vi "TestLauncher.vi"() -> ()   [LabVIEW 2020, in "ECU_Diagnose.lvlib"]
uses:
  ECU_Diagnose.lvlib
  SignalSenderLoop/SignalSenderLoop.lvclass
  C:/Program Files (x86)/National Instruments/LabVIEW 2020/vi.lib/JKI/JKI SMO/SMO/SMO.lvclass
  SignalReceiver/Typedefs/SignalArrySelecte.ctl
  SignalSenderLoop/subvi/SignalFrameSet.ctl
  SignalReceiver/GlobalData_operation.ctl
  SignalReceiver/SignalReceiver.lvclass
  <vilib>/JKI/JKI SMO/SMO/SMO.lvclass
  UDS_class/UDS.lvclass
  <vilib>/addons/_AddQ/G#Object/G#Object.lvclass
  <vilib>/Automotive Diagnostic Command Set/Diagnostic Transport.llb/Property ID.ctl
  <vilib>/addons/Automotive Diagnostic Command Set/NI_Automotive Diagnostic Command Set.lvlib
  <vilib>/Utility/config.llb/NI_LVConfig.lvlib
panel:
  in  "ClaerData":bool
  in  "Close":bool
  in  "总关闭":bool
  in  "信号收发参数":T3={"信号接收参数"={"Port_No."="CAN1", "XNET Signal"=[]}, "信号轮询发送参数"={"XNET SignalFrameArry"=[{"Port_No."="CAN1", "计数Count"=TRUE, "校验CheckSum"=TRUE, "MessageFrame"="ESP_1\nLR110", "校验算法名称"="Anti_Add"}, {"Port_No."="CAN1", "计数Count"=FALSE, "校验CheckSum"=FALSE, "MessageFrame"="VTOG_1\nLR110", "校验算法名称"=""}]}}
  in  "Save":bool
  in  "Read":bool
  out "DataIdentify":string
  out "Clear DTC":bool
  out "DID":u8[](array[numeric]) format="%.0x"
  out "OK":bool
  out "# of objects killed":i32
  out "Waveform Graph":dbl[][](graph)
  in  "StartStop":bool
  in  "Stop 2":bool
  out "error out":errorcluster
  out "数组":errorcluster[](array[cluster])
  in  "SignalsSet":dbl[](array[numeric])=[-32.0, 0.0, 1.0, 0.0, 1.0, 0.0, 1.0, 0.0, 1.0, 0.0, 1.0, 0.0, 1.0]
  in  "Stop":bool
  in  "SignalsSet 2":dbl[](array[numeric])=[0.0]
  out "元素":refnum<class "SignalSenderLoop.lvclass">
  out "SMOArry":refnum<class "SignalSenderLoop.lvclass">[](array[class])
  # "Signals Sender"
  # "数组为空，不发送任何帧，即停止发送\n首次运行时需要值改变触发一下"
  # "Signals Receiver"
  # "UDS Dignose Sender"
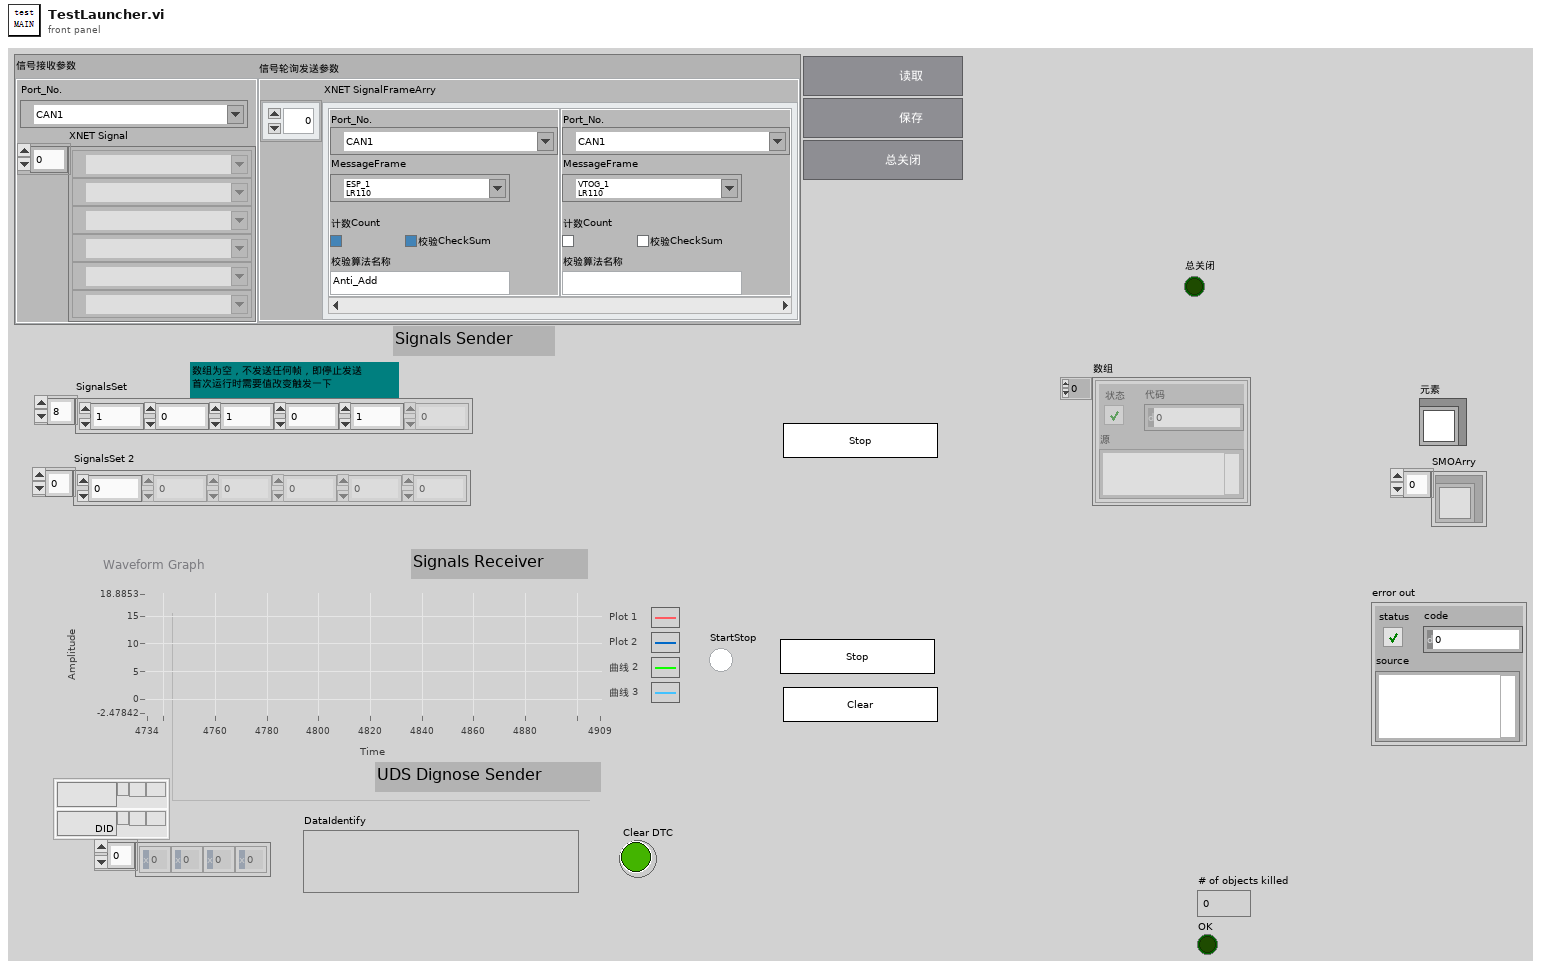
[diagram p1: front panel]
types:
  T1 = typedef "ECU_Diagnose.lvlib/SignalReceiver.lvclass/SignalArrySelecte.ctl" = cluster{"Port_No.":refnum<k21>, "XNET Signal":refnum<k21>[]}
  T2 = typedef "ECU_Diagnose.lvlib/SignalSenderLoop.lvclass/SignalFrameSet.ctl" = cluster{"Port_No.":refnum<k21>, "计数Count":bool, "校验CheckSum":bool, "MessageFrame":refnum<k21>, "校验算法名称":string}
  T3 = cluster{"信号接收参数":T1, "信号轮询发送参数":cluster{"XNET SignalFrameArry":T2[]}}
  T4 = typedef "GlobalData_operation.ctl" = enum16{"idle", "read", "write", "clear", "init", "destroy"}
  T5 = typedef "NI_Automotive Diagnostic Command Set.lvlib/Property ID.ctl" = enum16{"Timeout Diag Command", "Timeout FC (Bs)", "Timeout CF (Cr)", "Receive Block Size (BS)", "Wait Time CF (STmin)", "Max Wait Frames (N_WFTmax)", "Wait Frames to Send (N_WAIT)", "Time between Waits (T_W)", "Fill CAN Frames", "Fill Byte", "Invalid Response as Error", "Max RspPending Count", "VWTP Command Timeout", "STmin", "P2min", "Termination", "Timeout RspPending", "LIN Sleep", "Actual CAN IO Mode", "Response Plausibility Check", "Session-based Properties"}
  T6 = typedef "NI_LVConfig.lvlib/Config Data RefNum.ctl" = refnum<k1>
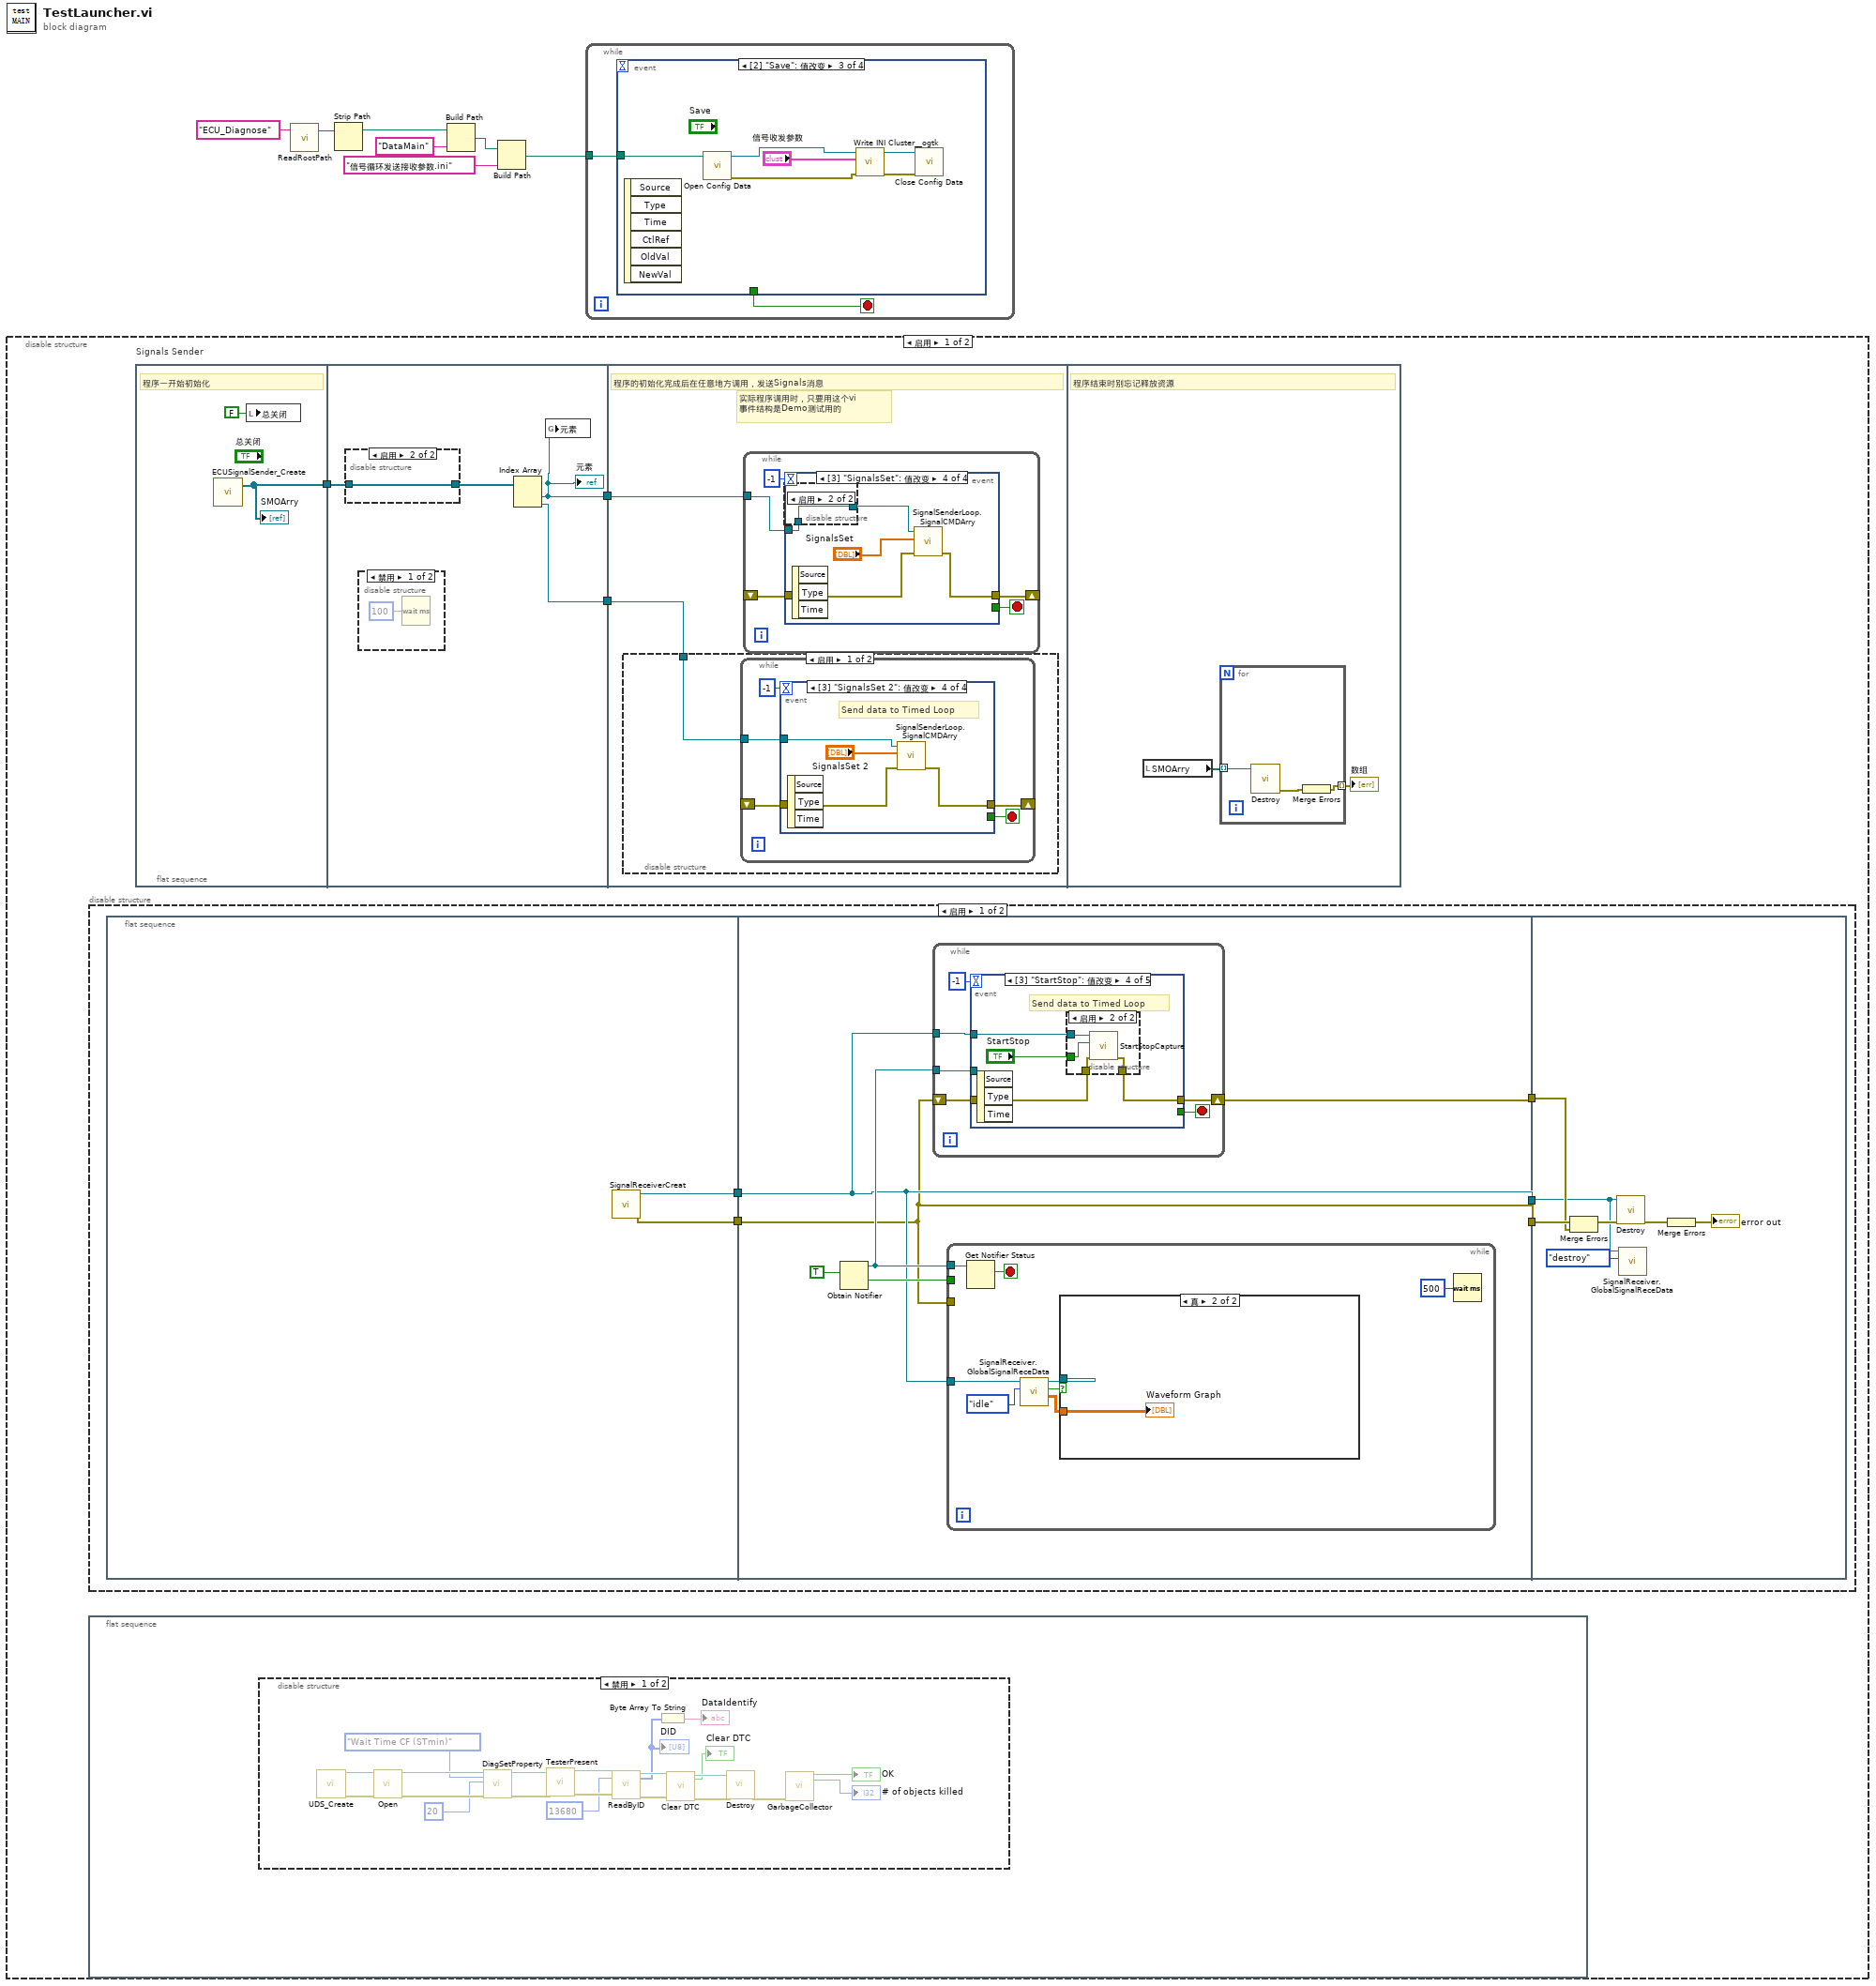
[diagram p0: block diagram]
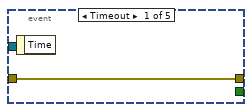
[diagram p3: hidden frame]
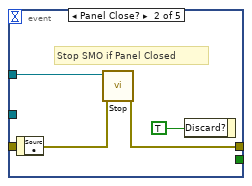
[diagram p4: hidden frame]
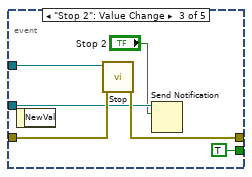
[diagram p5: hidden frame]
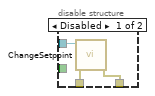
[diagram p6: hidden frame]
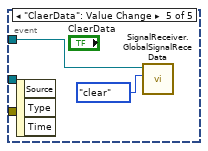
[diagram p7: hidden frame]
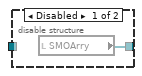
[diagram p10: hidden frame]
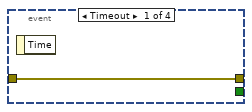
[diagram p12: hidden frame]
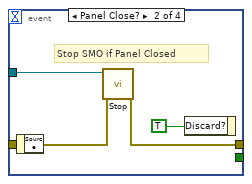
[diagram p13: hidden frame]
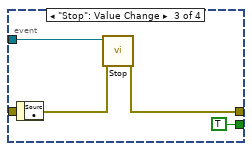
[diagram p14: hidden frame]
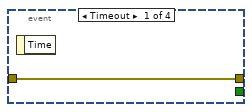
[diagram p16: hidden frame]
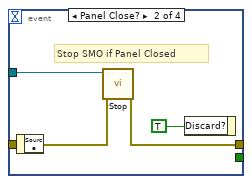
[diagram p17: hidden frame]
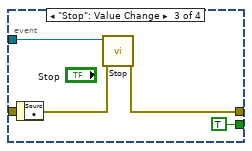
[diagram p18: hidden frame]
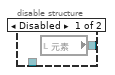
[diagram p19: hidden frame]
diagram:
  n1 = disable-structure shown="启用" {
    frame Enabled {
      n2 = flat-sequence {
        frame #0 {
          n3 = disable-structure shown="禁用" {
            frame Disabled {
              n4 = call "UDS_Create.vi"() -> ("reference out"=w90:refnum<class "UDS.lvclass">, "error out"=w89:errorcluster)  [unwired: 18 in]
              n5 = call-dynamic "Open.vi"("reference in"=w90, "error in (no error)"=w89) -> ("reference out"=w88:refnum<class "UDS.lvclass">, "error out"=w87:errorcluster)  [unwired: 16 in]
              n6 = call-dynamic "DiagSetProperty.vi"("reference in"=w88, "property ID"=Property_ID."Wait Time CF (STmin)", "property value"=u32 20, "error in (no error)"=w87) -> ("reference out"=w86:refnum<class "UDS.lvclass">, "error out"=w85:errorcluster)  [unwired: 14 in]
              n7 = call-dynamic "TesterPresent.vi"("reference in"=w86, "error in (no error)"=w85) -> ("reference out"=w84:refnum<class "UDS.lvclass">, "error out"=w83:errorcluster)  [unwired: 16 in]
              n8 = call-dynamic "ReadByID.vi"("reference in"=w84, "ID"=u16 13680, "error in (no error)"=w83) -> ("reference out"=w82:refnum<class "UDS.lvclass">, "DID"=w71:u8[], "error out"=w81:errorcluster)  [unwired: 14 in]
              "DID" <- w71
              n9 = Byte Array To String(unsigned byte array=w71) -> (string=→"DataIdentify":string)
              n10 = call-dynamic "Clear DTC.vi"("reference in"=w82, "error in (no error)"=w81) -> ("reference out"=w80:refnum<class "UDS.lvclass">, "Clear DTC"=→"Clear DTC":bool, "error out"=w79:errorcluster)  [unwired: 15 in]
              n11 = call-dynamic <vilib>:"Destroy.vi"("reference in"=w80, "error in (no error)"=w79) -> ("error out"=w76:errorcluster)  [unwired: 16 in, 1 out]
              n12 = call <vilib>:"GarbageCollector.vi"("error in (no error)"=w76) -> ("OK"=→"OK":bool, "# of objects killed"=→"# of objects killed":i32)  [unwired: 16 in, 1 out]
            }
            frame Enabled {
            }
          }
        }
      }
      n13 = disable-structure shown="启用" {
        frame Enabled {
          n14 = flat-sequence {
            tunnel: [w16] -> w15
            tunnel: [w17] -> w14
            tunnel: [w19] -> w13
            tunnel: [w18] -> w12
            tunnel: [w20] -> w11
            tunnel: w15 -> [w18]
            tunnel: w14 -> [w19]
            tunnel: w13 -> [w64]
            tunnel: w12 -> [w66]
            tunnel: w11 -> [w65]
            frame #0 {
              n15 = call "SignalReceiverCreat.vi"() -> ("SignalReceiver out"=w17:refnum<class "SignalReceiver.lvclass">, "错误输出"=w16:errorcluster)  [unwired: 17 in, 1 out]
            }
            frame #1 {
              n16 = Obtain Notifier(notification data type=TRUE) -> (notifier out=w21:refnum<notifier>, created new?=w22:bool)  [unwired: 3 in, 1 out]
              n17 = while {
                shift-right: [w37] -> w20
                shift-left: w18 -> [w36]
                tunnel: w21 -> [w34]
                tunnel: w19 -> [w33]
                stop <- w38 stop-if-true
                n18 = event shown="[3] \"StartStop\": 值改变" {
                  selector: _ -> [_ _ _ _ _]
                  dyn-events: _ -> [_ _ _ _ _]
                  timeout: -1 -> [_ _ _ _ _]
                  tunnel: [_ _ TRUE _ _] -> w38
                  tunnel: w33 -> [_ w43 w49 w53 w61]
                  tunnel: [w39 w42 w48 w51 _] -> w37
                  tunnel: w36 -> [w39 w41 w47 w52 _]
                  tunnel: w34 -> [_ _ w46 _ _]
                  event Timeout {
                    n19 = event-data() -> ()  [unwired: 1 in, 1 out]
                  }
                  event Panel Close? {
                    # "Stop SMO if Panel Closed"
                    n20 = event-data() -> ()  [unwired: 1 in, 1 out]
                    n21 = call <vilib>:"Stop.vi"("error in (no error)"=w41, "SMO"=w43) -> ("error out"=w42:errorcluster)  [unwired: 8 in, 1 out]
                    n22 = event-data("Discard?"=TRUE ("OK")) -> ()  [unwired: 1 in, 1 out]
                  }
                  event "Stop 2": Value Change {
                    n23 = event-data() -> ()  [unwired: 1 in, 1 out]
                    n24 = call <vilib>:"Stop.vi"("error in (no error)"=w47, "SMO"=w49) -> ("error out"=w48:errorcluster)  [unwired: 8 in, 1 out]
                    n25 = Send Notification(notification="Stop 2", notifier=w46) -> ()  [unwired: 1 in, 2 out]
                  }
                  event "StartStop": Value Change {
                    # "Send data to Timed Loop"
                    n26 = event-data() -> ()  [unwired: 1 in, 3 out]
                    n27 = disable-structure shown="启用" {
                      disable-tunnel: w53 -> [w56 w60]
                      disable-tunnel: w52 -> [w55 w59]
                      disable-tunnel: [w54 w58] -> w51
                      disable-tunnel: "StartStop" -> [_ w57]
                      frame Disabled {
                        n28 = call "ChangeSetpoint.vi"("error in (no error)"=w55, "SignalReceiver"=w56) -> ("error out"=w54:errorcluster)  [unwired: 8 in, 1 out]
                      }
                      frame Enabled {
                        n29 = call "StartStopCapture.vi"("error in (no error)"=w59, "StartStopCapture"=w57, "SignalReceiver"=w60) -> ("error out"=w58:errorcluster)  [unwired: 7 in, 1 out]
                      }
                    }
                  }
                  event "ClaerData": Value Change {
                    n30 = event-data() -> ()  [unwired: 1 in, 3 out]
                    n31 = call "SignalReceiver.GlobalSignalReceData.vi"("operation"=GlobalData_operation."clear", "SignalReceiver"=w61) -> ()  [unwired: 6 in, 4 out]
                  }
                }
              }
              n32 = while {
                tunnel: w18 -> [_]
                tunnel: w19 -> [w28]
                tunnel: w22 -> [_]
                tunnel: w21 -> [w26]
                stop <- w25 stop-if-true
                n33 = Get Notifier Status(notifier=w26) -> (current notification=w25:bool)  [unwired: 1 in, 4 out]
                n34 = call "SignalReceiver.GlobalSignalReceData.vi"("operation"=GlobalData_operation."idle", "SignalReceiver"=w28) -> ("SignalDatOut"=w24:dbl[][], "Update"=w29:bool, "SignalReceiver out"=w27:refnum<class "SignalReceiver.lvclass">)  [unwired: 6 in, 1 out]
                n35 = case shown="真" w29 {
                  tunnel: w27 -> [_ _]
                  tunnel: w24 -> [_ w32]
                  frame False {
                  }
                  frame True {
                    "Waveform Graph" <- w32
                  }
                }
                n36 = Wait (ms)(milliseconds to wait=u32 500 ("等待时间（毫秒）")) -> ()  [unwired: 1 out]
              }
            }
            frame #2 {
              n37 = Merge Errors(w66, w65) -> (w69:errorcluster)
              n38 = call <vilib>:"Destroy.vi"("error in (no error)"=w69, "SMO"=w64) -> ("error out"=w68:errorcluster)  [unwired: 9 in]
              n39 = call "SignalReceiver.GlobalSignalReceData.vi"("operation"=GlobalData_operation."destroy", "SignalReceiver"=w64) -> ()  [unwired: 6 in, 4 out]
              n40 = Merge Errors(w68) -> (→"error out":errorcluster)
            }
          }
        }
        frame Disabled {
        }
      }
      n41 = flat-sequence "Signals Sender" {
        tunnel: [w92] -> w10
        tunnel: [w94] -> w9
        tunnel: [w95] -> w8
        tunnel: w10 -> [w93]
        tunnel: w9 -> [w101]
        tunnel: w8 -> [w100]
        frame #0 {
          # "程序一开始初始化"
          n42 = call "ECUSignalSender_Create.vi"() -> ("SMOArry"=w92:refnum<class "SignalSenderLoop.lvclass">[])  [unwired: 17 in, 2 out]
          "SMOArry" <- w92
          n43 = local write "总关闭"(FALSE ("总关闭")) -> ()
        }
        frame #1 {
          n44 = disable-structure shown="启用" {
            disable-tunnel: [w97 w98] -> w96
            disable-tunnel: w93 -> [_ w98]
            frame Disabled {
              n45 = local read "SMOArry"() -> (w97:refnum<class "SignalSenderLoop.lvclass">[])
            }
            frame Enabled {
            }
          }
          n46 = disable-structure shown="禁用" {
            frame Disabled {
              n47 = Wait (ms)(milliseconds to wait=u32 100 ("等待时间（毫秒）")) -> ()  [unwired: 1 out]
            }
            frame Enabled {
            }
          }
          n48 = Index Array(array=w96) -> (element #1=w94:refnum<class "SignalSenderLoop.lvclass">, element #2=w95:refnum<class "SignalSenderLoop.lvclass">)  [unwired: 2 in]
          "元素" <- w94
          n49 = global write "test 1.vi" "元素"(w94) -> ()
        }
        frame #2 {
          # "实际程序调用时，只要用这个vi\n事件结构是Demo测试用的"
          # "程序的初始化完成后在任意地方调用，发送Signals消息"
          n50 = disable-structure shown="启用" {
            disable-tunnel: w100 -> [w102 _]
            frame Enabled {
              n51 = while {
                shift-right: [w106] -> _
                shift-left: _ -> [w105]
                tunnel: w102 -> [w104]
                stop <- w107 stop-if-true
                n52 = event shown="[3] \"SignalsSet 2\": 值改变" {
                  selector: _ -> [_ _ _ _]
                  dyn-events: _ -> [_ _ _ _]
                  timeout: -1 -> [_ _ _ _]
                  tunnel: [_ _ TRUE _] -> w107
                  tunnel: w104 -> [_ w112 w116 w120]
                  tunnel: [w108 w111 w115 w117] -> w106
                  tunnel: w105 -> [w108 w110 w114 w118]
                  event Timeout {
                    n53 = event-data() -> ()  [unwired: 1 in, 1 out]
                  }
                  event Panel Close? {
                    # "Stop SMO if Panel Closed"
                    n54 = event-data() -> ()  [unwired: 1 in, 1 out]
                    n55 = call <vilib>:"Stop.vi"("error in (no error)"=w110, "SMO"=w112) -> ("error out"=w111:errorcluster)  [unwired: 8 in, 1 out]
                    n56 = event-data("Discard?"=TRUE ("OK")) -> ()  [unwired: 1 in, 1 out]
                  }
                  event "Stop": Value Change {
                    n57 = event-data() -> ()  [unwired: 1 in, 1 out]
                    n58 = call <vilib>:"Stop.vi"("error in (no error)"=w114, "SMO"=w116) -> ("error out"=w115:errorcluster)  [unwired: 8 in, 1 out]
                  }
                  event "SignalsSet 2": Value Change {
                    # "Send data to Timed Loop"
                    n59 = event-data() -> ()  [unwired: 1 in, 3 out]
                    n60 = call "SignalSenderLoop.SignalCMDArry.vi"("error in (no error)"=w118, "SignalCMDArry"="SignalsSet 2", "SignalSenderLoop"=w120) -> ("error out"=w117:errorcluster)  [unwired: 7 in, 1 out]
                  }
                }
              }
            }
            frame Disabled {
            }
          }
          n61 = while {
            shift-right: [w124] -> _
            shift-left: _ -> [w123]
            tunnel: w101 -> [w121]
            stop <- w125 stop-if-true
            n62 = event shown="[3] \"SignalsSet\": 值改变" {
              selector: _ -> [_ _ _ _]
              dyn-events: _ -> [_ _ _ _]
              timeout: -1 -> [_ _ _ _]
              tunnel: [_ _ TRUE _] -> w125
              tunnel: [w126 w130 w134 w138] -> w124
              tunnel: w123 -> [w126 w129 w133 w139]
              tunnel: w121 -> [_ w127 w132 w135]
              event Timeout {
                n63 = event-data() -> ()  [unwired: 1 in, 1 out]
              }
              event Panel Close? {
                # "Stop SMO if Panel Closed"
                n64 = event-data() -> ()  [unwired: 1 in, 1 out]
                n65 = call <vilib>:"Stop.vi"("error in (no error)"=w129, "SMO"=w127) -> ("error out"=w130:errorcluster)  [unwired: 8 in, 1 out]
                n66 = event-data("Discard?"=TRUE ("OK")) -> ()  [unwired: 1 in, 1 out]
              }
              event "Stop": Value Change {
                n67 = event-data() -> ()  [unwired: 1 in, 1 out]
                n68 = call <vilib>:"Stop.vi"("error in (no error)"=w133, "SMO"=w132) -> ("error out"=w134:errorcluster)  [unwired: 8 in, 1 out]
              }
              event "SignalsSet": Value Change {
                n69 = disable-structure shown="启用" {
                  disable-tunnel: [w140 w141] -> w136
                  disable-tunnel: w135 -> [_ w141]
                  frame Disabled {
                    n70 = local read "元素"() -> (w140:refnum<class "SignalSenderLoop.lvclass">)
                  }
                  frame Enabled {
                  }
                }
                n71 = event-data() -> ()  [unwired: 1 in, 3 out]
                n72 = call "SignalSenderLoop.SignalCMDArry.vi"("error in (no error)"=w139, "SignalCMDArry"="SignalsSet", "SignalSenderLoop"=w136) -> ("error out"=w138:errorcluster)  [unwired: 7 in, 1 out]
              }
            }
          }
        }
        frame #3 {
          # "程序结束时别忘记释放资源"
          n73 = local read "SMOArry"() -> (w142:refnum<class "SignalSenderLoop.lvclass">[])
          n74 = for {
            tunnel: [w145] -> w143 mode=indexing
            tunnel: w142 -> [w144] mode=indexing
            n75 = call <vilib>:"Destroy.vi"("SMO"=w144) -> ("error out"=w146:errorcluster)  [unwired: 10 in]
            n76 = Merge Errors(w146) -> (w145:errorcluster)
          }
          "数组" <- w143
        }
      }
    }
    frame Disabled {
    }
  }
  n77 = call "ReadRootPath.vi"("BuildRootFolder"="ECU_Diagnose" ("ConfigFlieFolderName")) -> ("Root path"=w3:path)  [unwired: 18 in]
  n78 = Strip Path(path=w3) -> (stripped path=w2:path)  [unwired: 1 out]
  n79 = Build Path(base path=w2, name or relative path="DataMain" ("ConfigFlieFolderName")) -> (appended path=w7:path)
  n80 = Build Path(base path=w7, name or relative path="信号循环发送接收参数.ini" ("ConfigFlieFolderName")) -> (appended path=w1:path)
  n81 = while {
    tunnel: w1 -> [w147]
    stop <- w148 stop-if-true
    n82 = event shown="[2] \"Save\": 值改变" {
      selector: _ -> [_ _ _ _]
      dyn-events: _ -> [_ _ _ _]
      timeout: _ -> [_ _ _ _]
      tunnel: [_ _ _ w163] -> w148
      tunnel: w147 -> [_ w151 w159 _]
      event Timeout {
        n83 = event-data() -> ()  [unwired: 1 in, 3 out]
      }
      event "Read": Value Change {
        n84 = event-data() -> ()  [unwired: 1 in, 6 out]
        n85 = local read "信号收发参数"() -> (w154:T3)
        n86 = call <vilib>:"Open Config Data.vi"("configuration file path"=w151) -> ("error out"=w149:errorcluster, "refnum"=w150:T6)  [unwired: 8 in, 1 out]
        n87 = call <userlib>:"Read INI Cluster__ogtk.vi"("error in (no error)"=w149, "INI Fomatted Cluster Type"=w154, "refnum"=w150) -> ("error out"=w152:errorcluster, "INI Fomatted Cluster"=w156:variant, "dup refnum"=w153:T6)  [unwired: 4 in, 2 out]
        n88 = Variant To Data(type=w154, Variant=w156) -> (data=w155:T3)  [unwired: 1 in, 1 out]
        n89 = local write "信号收发参数"(w155) -> ()
        n90 = call <vilib>:"Close Config Data.vi"("error in (no error)"=w152, "refnum"=w153) -> ()  [unwired: 8 in, 2 out]
      }
      event "Save": Value Change {
        n91 = event-data() -> ()  [unwired: 1 in, 6 out]
        n92 = call <vilib>:"Open Config Data.vi"("configuration file path"=w159) -> ("error out"=w157:errorcluster, "refnum"=w158:T6)  [unwired: 8 in, 1 out]
        n93 = call <userlib>:"Write INI Cluster__ogtk.vi"("error in (no error)"=w157, "INI Fomatted Cluster"="信号收发参数", "refnum"=w158) -> ("error out"=w160:errorcluster, "dup refnum"=w161:T6)  [unwired: 7 in]
        n94 = call <vilib>:"Close Config Data.vi"("error in (no error)"=w160, "refnum"=w161) -> ()  [unwired: 8 in, 2 out]
      }
      event "Close": Value Change {
        n95 = event-data() -> ("NewVal"=w163:bool)  [unwired: 1 in, 5 out]
      }
    }
  }
